vi "44xx_AO_MinMax.vi"(9 "AO.channels":tag, 10 "AO.Range":T1) -> (1 "ProductType":string, 2 "AO.max":dbl, 3 "AO.min":dbl)   [LabVIEW 2016, in "LockinDAQ.lvclass"]
uses:
  LockinDAQ.lvclass
  Typedefs/446xAO-enum.ctl
  <resource>/objmgr/daqmx.rc
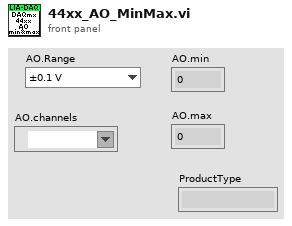
[diagram p1: front panel]
types:
  T1 = typedef "446xAO-enum.ctl" = enum16{"±0.1 V", "±1.0 V", "±10.0 V"}
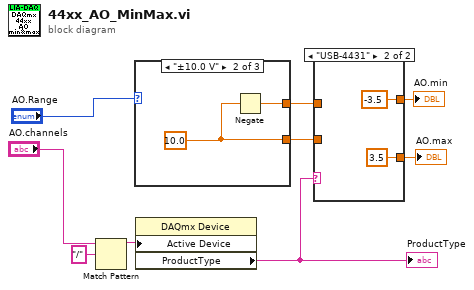
[diagram p0: block diagram]
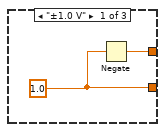
[diagram p3: hidden frame]
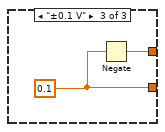
[diagram p4: hidden frame]
diagram:
  n1 = Match Pattern(string="AO.channels", regular expression="/") -> (before substring=w8:string)  [unwired: 1 in, 3 out]
  n2 = case shown="\"±10.0 V\"" "AO.Range" {
    tunnel: [w11 w13 w15] -> w1
    tunnel: [w10 w12 w14] -> w3
    frame "±1.0 V" {
      w11 = 1.0
      n3 = Negate(x=w11) -> (-x=w10:dbl)
    }
    frame "±10.0 V" {
      w13 = 10.0
      n4 = Negate(x=w13) -> (-x=w12:dbl)
    }
    frame "±0.1 V" {
      w15 = 0.1
      n5 = Negate(x=w15) -> (-x=w14:dbl)
    }
  }
  n6 = property class="DAQmx Device"("Active Device"=w8) -> ("ProductType"=w5:string)  [unwired: 2 in, 2 out]
  "ProductType" <- w5
  n7 = case shown="\"USB-4431\"" w5 {
    tunnel: [w17 -3.5] -> w4
    tunnel: w3 -> [w17 _]
    tunnel: [w16 3.5] -> w2
    tunnel: w1 -> [w16 _]
    frame "", Default {
    }
    frame "USB-4431" {
    }
  }
  "AO.min" <- w4
  "AO.max" <- w2
